vi "getAdditionalDataXML.vi"(8 "error in (no error)":errorcluster, 11 "RfRamp in":refnum<class "RfRamp.lvclass">) -> (0 "error out":errorcluster, 2 "additionalDataXML":refnum<class "xmlNode.lvclass">, 3 "RfRamp out":refnum<class "RfRamp.lvclass">)   [LabVIEW 2011, in "Tools.lvlib" / "Scripting.lvlib" / "RfRamp.lvclass"]
uses:
  RfRamp.lvclass
  xmlNode/xmlNode.lvclass
  RfRamp.lvclass/RfRamp.ctl
  ScriptEvent.lvclass
  Rf Event/rf.lvclass
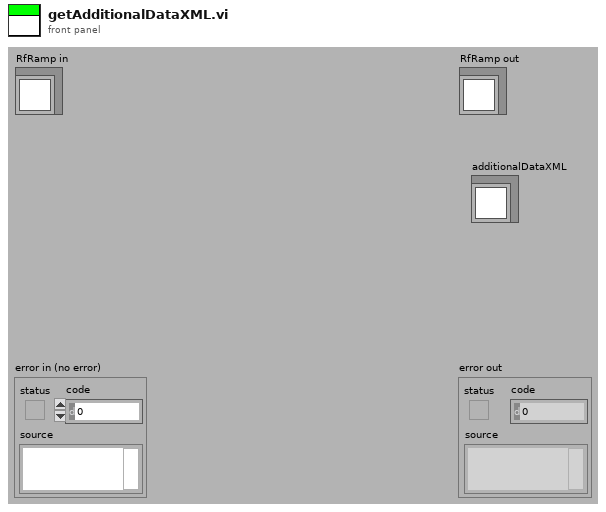
[diagram p1: front panel]
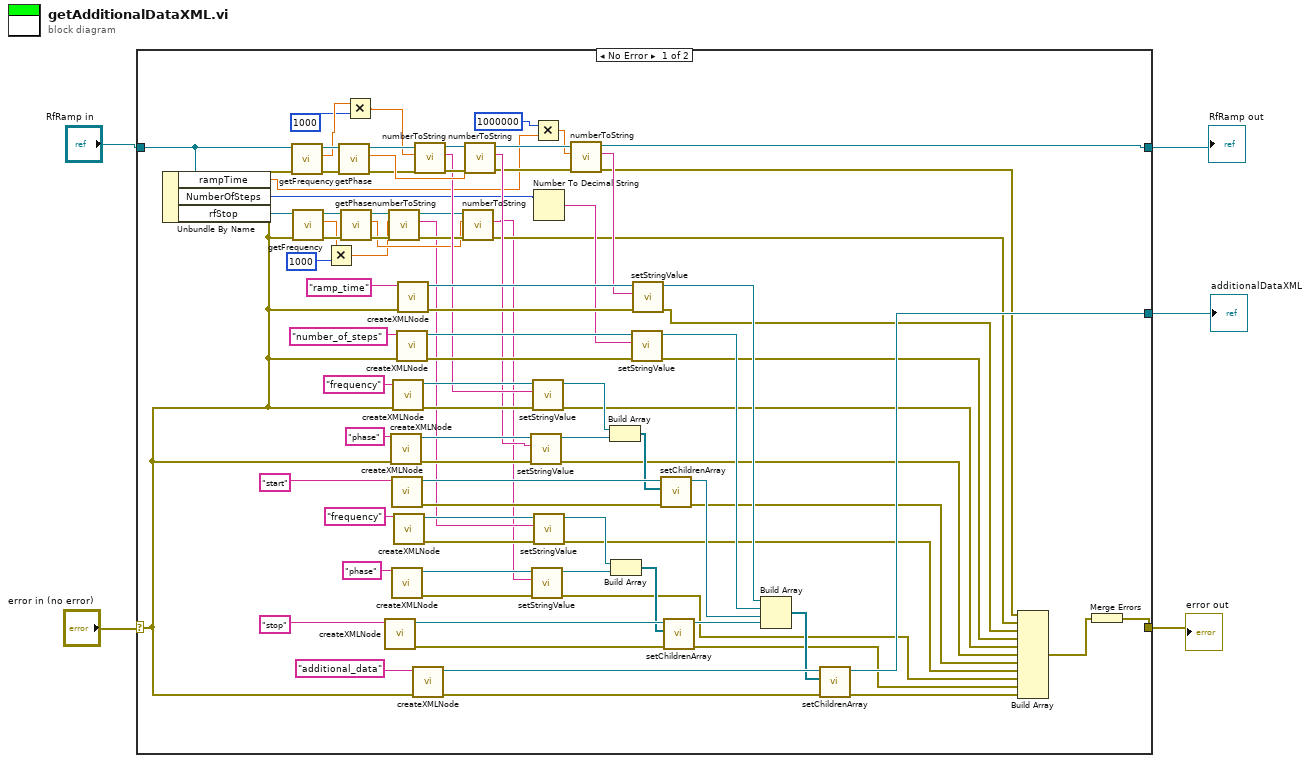
[diagram p0: block diagram]
diagram:
  n1 = case shown="No Error" "error in (no error)" {
    selector: "error in (no error)" -> [w71 w94]
    tunnel: [w19 w94] -> w3
    tunnel: [w17 w95] -> w1
    tunnel: "RfRamp in" -> [w79 w95]
    tunnel: [w86 _] -> w2
    frame No Error {
      n2 = Unbundle By Name(w79) -> ("rampTime"=w7:dbl, "NumberOfSteps"=w49:i32, "rfStop"=w78:refnum<class "rf.lvclass">)
      n3 = call "getFrequency.vi"("error in (no error)"=w71, "rf in"=w79) -> ("error out"=w64:errorcluster, "frequency"=w14:dbl, "rf out"=w65:refnum<class "RfRamp.lvclass">)  [unwired: 7 in]
      n4 = call "getFrequency.vi"("error in (no error)"=w71, "rf in"=w78) -> ("error out"=w57:errorcluster, "frequency"=w11:dbl, "rf out"=w58:refnum<class "rf.lvclass">)  [unwired: 7 in]
      n5 = Multiply(x=w11, y=1000) -> (x*y=w10:dbl)
      n6 = call "getPhase.vi"("error in (no error)"=w64, "rf in"=w65) -> ("error out"=w61:errorcluster, "phase"=w63:dbl, "rf out"=w62:refnum<class "RfRamp.lvclass">)  [unwired: 7 in]
      n7 = call "getPhase.vi"("error in (no error)"=w57, "rf in"=w58) -> ("error out"=w53:errorcluster, "phase"=w52:dbl, "rf out"=w54:refnum<class "rf.lvclass">)  [unwired: 7 in]
      n8 = Multiply(x=w14, y=1000) -> (x*y=w12:dbl)
      n9 = call "createXMLNode.vi"("name"="stop") -> ("error out"=w37:errorcluster, "xmlNode out"=w38:refnum<class "xmlNode.lvclass">)  [unwired: 9 in]
      n10 = call "numberToString.vi"("error in (no error)"=w53, "Numeric"=w10, "ScriptEvent in"=w54) -> ("error out"=w56:errorcluster, "String"=w16:string, "ScriptEvent out"=w55:refnum<class "rf.lvclass">)  [unwired: 6 in]
      n11 = call "createXMLNode.vi"("error in (no error)"=w71, "name"="phase") -> ("error out"=w83:errorcluster, "xmlNode out"=w84:refnum<class "xmlNode.lvclass">)  [unwired: 8 in]
      n12 = call "createXMLNode.vi"("name"="start") -> ("error out"=w67:errorcluster, "xmlNode out"=w68:refnum<class "xmlNode.lvclass">)  [unwired: 9 in]
      n13 = call "createXMLNode.vi"("name"="phase") -> ("error out"=w40:errorcluster, "xmlNode out"=w41:refnum<class "xmlNode.lvclass">)  [unwired: 9 in]
      n14 = call "createXMLNode.vi"("error in (no error)"=w71, "name"="frequency") -> ("error out"=w91:errorcluster, "xmlNode out"=w92:refnum<class "xmlNode.lvclass">)  [unwired: 8 in]
      n15 = call "createXMLNode.vi"("name"="frequency") -> ("error out"=w44:errorcluster, "xmlNode out"=w45:refnum<class "xmlNode.lvclass">)  [unwired: 9 in]
      n16 = call "createXMLNode.vi"("error in (no error)"=w71, "name"="number_of_steps") -> ("error out"=w73:errorcluster, "xmlNode out"=w74:refnum<class "xmlNode.lvclass">)  [unwired: 8 in]
      n17 = call "createXMLNode.vi"("error in (no error)"=w71, "name"="ramp_time") -> ("error out"=w76:errorcluster, "xmlNode out"=w77:refnum<class "xmlNode.lvclass">)  [unwired: 8 in]
      n18 = call "createXMLNode.vi"("error in (no error)"=w71, "name"="additional_data") -> ("error out"=w88:errorcluster, "xmlNode out"=w90:refnum<class "xmlNode.lvclass">)  [unwired: 8 in]
      n19 = call "numberToString.vi"("error in (no error)"=w61, "Numeric"=w12, "ScriptEvent in"=w62) -> ("error out"=w82:errorcluster, "String"=w60:string, "ScriptEvent out"=w81:refnum<class "RfRamp.lvclass">)  [unwired: 6 in]
      n20 = call "numberToString.vi"("error in (no error)"=w56, "Numeric"=w52, "ScriptEvent in"=w55) -> ("error out"=w21:errorcluster, "String"=w15:string)  [unwired: 6 in, 1 out]
      n21 = call "numberToString.vi"("error in (no error)"=w82, "Numeric"=w63, "ScriptEvent in"=w81) -> ("error out"=w50:errorcluster, "String"=w59:string, "ScriptEvent out"=w51:refnum<class "RfRamp.lvclass">)  [unwired: 6 in]
      n22 = call-dynamic "setStringValue.vi"("error in (no error)"=w83, "stringValue"=w59, "xmlNode.lvclass in"=w84) -> ("error out"=w25:errorcluster, "xmlNode.lvclass out"=w80:refnum<class "xmlNode.lvclass">)  [unwired: 7 in]
      n23 = call-dynamic "setStringValue.vi"("error in (no error)"=w40, "stringValue"=w15, "xmlNode.lvclass in"=w41) -> ("error out"=w28:errorcluster, "xmlNode.lvclass out"=w39:refnum<class "xmlNode.lvclass">)  [unwired: 7 in]
      n24 = Multiply(x=1000000, y=w7) -> (x*y=w6:dbl)
      n25 = call-dynamic "setStringValue.vi"("error in (no error)"=w91, "stringValue"=w60, "xmlNode.lvclass in"=w92) -> ("error out"=w24:errorcluster, "xmlNode.lvclass out"=w87:refnum<class "xmlNode.lvclass">)  [unwired: 7 in]
      n26 = Number To Decimal String(number=w49) -> (decimal integer string=w48:string)  [unwired: 1 in]
      n27 = call-dynamic "setStringValue.vi"("error in (no error)"=w44, "stringValue"=w16, "xmlNode.lvclass in"=w45) -> ("error out"=w27:errorcluster, "xmlNode.lvclass out"=w43:refnum<class "xmlNode.lvclass">)  [unwired: 7 in]
      n28 = call "numberToString.vi"("error in (no error)"=w50, "Numeric"=w6, "ScriptEvent in"=w51) -> ("error out"=w20:errorcluster, "String"=w47:string, "ScriptEvent out"=w17:refnum<class "RfRamp.lvclass">)  [unwired: 6 in]
      n29 = Build Array(w87, w80) -> (w66:refnum<class "xmlNode.lvclass">[])
      n30 = Build Array(w43, w39) -> (w36:refnum<class "xmlNode.lvclass">[])
      n31 = call-dynamic "setStringValue.vi"("error in (no error)"=w73, "stringValue"=w48, "xmlNode.lvclass in"=w74) -> ("error out"=w23:errorcluster, "xmlNode.lvclass out"=w34:refnum<class "xmlNode.lvclass">)  [unwired: 7 in]
      n32 = call-dynamic "setStringValue.vi"("error in (no error)"=w76, "stringValue"=w47, "xmlNode.lvclass in"=w77) -> ("error out"=w22:errorcluster, "xmlNode.lvclass out"=w35:refnum<class "xmlNode.lvclass">)  [unwired: 7 in]
      n33 = call-dynamic "setChildrenArray.vi"("error in (no error)"=w67, "Children"=w66, "xmlNode.lvclass in"=w68) -> ("error out"=w26:errorcluster, "xmlNode.lvclass out"=w33:refnum<class "xmlNode.lvclass">)  [unwired: 7 in]
      n34 = call-dynamic "setChildrenArray.vi"("error in (no error)"=w37, "Children"=w36, "xmlNode.lvclass in"=w38) -> ("error out"=w29:errorcluster, "xmlNode.lvclass out"=w32:refnum<class "xmlNode.lvclass">)  [unwired: 7 in]
      n35 = Build Array(w35, w34, w33, w32) -> (w31:refnum<class "xmlNode.lvclass">[])
      n36 = call-dynamic "setChildrenArray.vi"("error in (no error)"=w88, "Children"=w31, "xmlNode.lvclass in"=w90) -> ("error out"=w30:errorcluster, "xmlNode.lvclass out"=w86:refnum<class "xmlNode.lvclass">)  [unwired: 7 in]
      n37 = Build Array(w20, w21, w22, w23, w24, w25, w26, w27, w28, w29, w30) -> (w18:errorcluster[])
      n38 = Merge Errors(w18) -> (w19:errorcluster)
    }
    frame Error {
    }
  }
  "error out" <- w3
  "RfRamp out" <- w1
  "additionalDataXML" <- w2
